vi "pp_writeClick.vi"(7 "Waveform Properties":T1={"Fs (Hz)"=20000.0, "Amplitude (V)"=5.0, "Ramp (s)"=0.005, "Duration (s)"=0.25} {"Ramp (s)" min=0.0; "Fs (Hz)" min=0.0}, 8 "Error In":errorcluster, 11 "DAQmx Analog Out In":refnum<k21>) -> (0 "Error Out":errorcluster, 2 "Waveform Out":waveform(dbl)={"t0"=timestamp(0 s since 1904-01-01), "dt"=5e-05, "Y"=array[5000 elements]}, 3 "DAQmx Analog Out Out":refnum<k21>)   [LabVIEW 2013]
uses:
  <vilib>/DAQmx/configure/timing.llb/DAQmx Timing (Use Waveform).vi
  <vilib>/DAQmx/write.llb/DAQmx Write (Analog Wfm 1Chan NSamp).vi
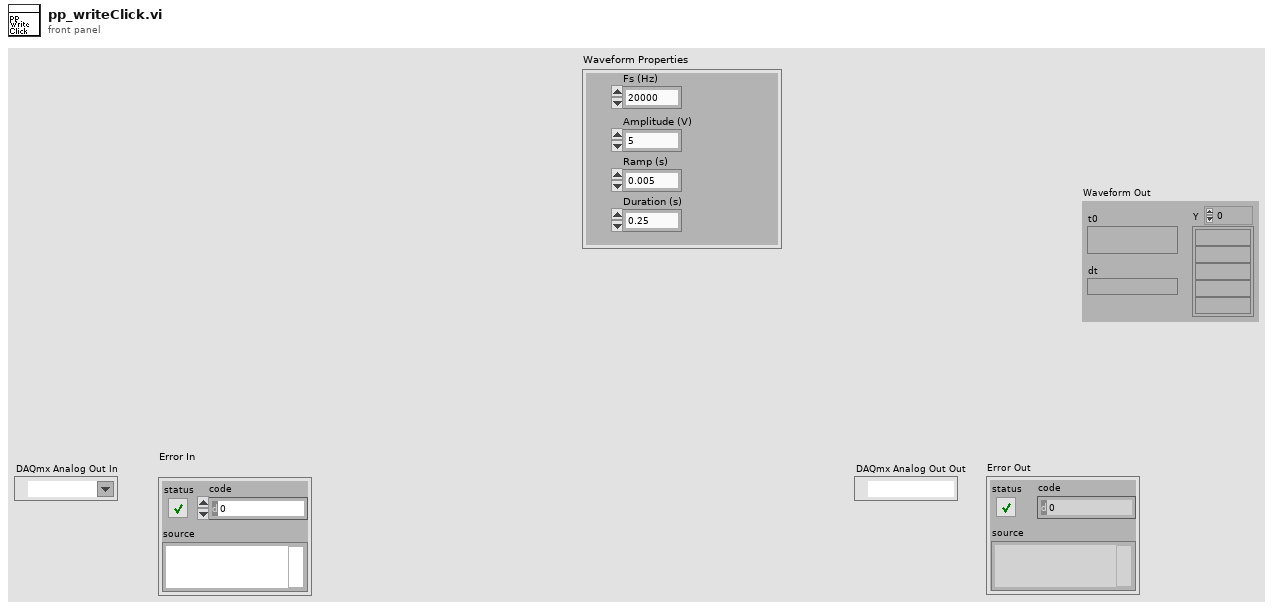
[diagram p1: front panel]
types:
  T1 = cluster{"Fs (Hz)":dbl, "Amplitude (V)":dbl, "Ramp (s)":dbl, "Duration (s)":dbl}
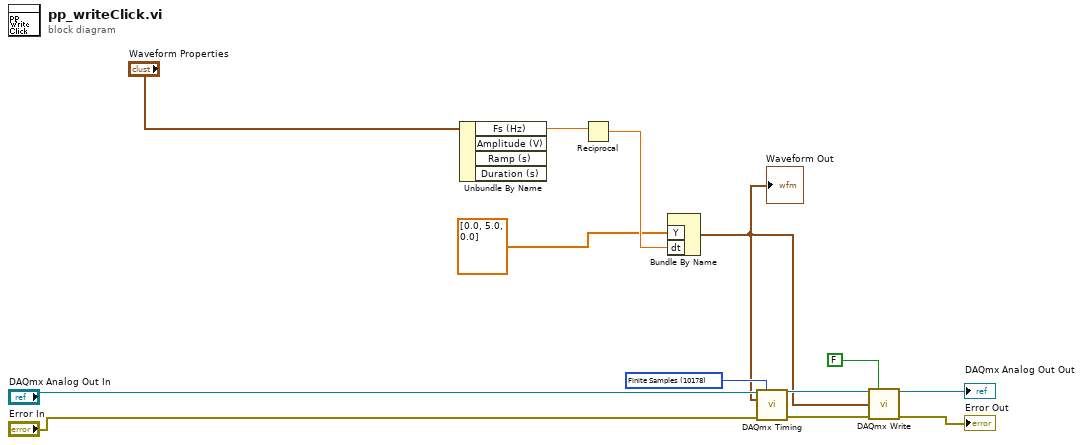
[diagram p0: block diagram]
diagram:
  w10 = 10178 items=["Finite Samples"=10178, "Continuous Samples"=10123, "Hardware Timed Single Point"=12522] ("sample mode")
  n1 = Unbundle By Name("Waveform Properties") -> ("Fs (Hz)"=w5:dbl)  [unwired: 3 out]
  n2 = Reciprocal(x=w5) -> (1/x=w4:dbl)
  n3 = Bundle By Name("Y"=dbl[] [0.0, 5.0, 0.0], "dt"=w4) -> (w2:waveform(dbl))  [unwired: 1 in]
  "Waveform Out" <- w2
  n4 = call-poly <vilib>:"DAQmx Timing.vi"("task/channels in"="DAQmx Analog Out In", "sample mode"=w10, "waveform"=w2, "error in"="Error In") -> ("task out"=w9:refnum<k21>, "error out"=w8:errorcluster)  [unwired: 10 in]
  n5 = call-poly <vilib>:"DAQmx Write.vi"("task/channels in"=w9, "auto start"=FALSE, "data"=w2, "error in"=w8) -> ("task out"=→"DAQmx Analog Out Out":refnum<k21>, "error out"=→"Error Out":errorcluster)  [unwired: 9 in, 1 out]
